vi "FindPropertyValue.vi"(7 "max len":i32=30, 10 "property":string, 11 "rows":string) -> (3 "value":string)   [LabVIEW 2020]
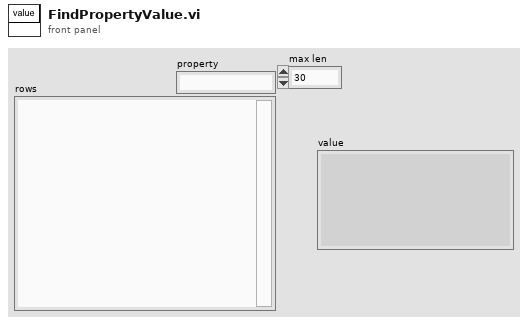
[diagram p1: front panel]
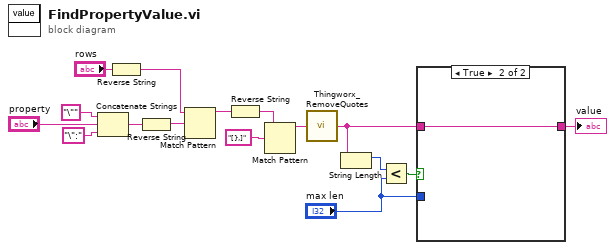
[diagram p0: block diagram]
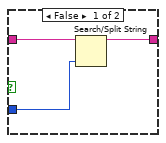
[diagram p2: hidden frame]
diagram:
  n1 = Concatenate Strings("\"" ("string"), "property", "\":" ("string")) -> (w13:string)
  n2 = Reverse String(1:"rows") -> (0:w9:string)
  n3 = Reverse String(1:w13) -> (0:w8:string)
  n4 = Match Pattern(string=w9, regular expression=w8) -> (before substring=w7:string)  [unwired: 1 in, 3 out]
  n5 = Reverse String(1:w7) -> (0:w6:string)
  n6 = Match Pattern(string=w6, regular expression="[},]") -> (before substring=w15:string)  [unwired: 1 in, 3 out]
  n7 = call "Thingworx_RemoveQuotes.vi"("Incoming string in"=w15) -> ("Incoming string out"=w4:string)
  n8 = String Length(string=w4) -> (length=w3:i32)
  n9 = Less?(x=w3, y="max len") -> (x < y?=w1:bool)
  n10 = case shown="True" w1 {
    tunnel: [w18 w20] -> w5
    tunnel: w4 -> [w19 w20]
    tunnel: "max len" -> [w17 _]
    frame False {
      n11 = Search/Split String(string=w19, offset (0)=w17) -> (substring before match=w18:string)  [unwired: 1 in, 2 out]
    }
    frame True {
    }
  }
  "value" <- w5
